vi "0516205_鍾禾翊_HW3.vi"() -> ()   [LabVIEW 2018]
panel:
  in  "Path to JPEG file":path=path "Afu.jpg"
  in  "stop 2":bool
  in  "stop":bool
  out "new picture 5":picture
  in  "Probe":dbl(slide) scale=0.0..10.0
  out "new picture 4":picture
  out "Brighten Image":picture
  out "Original Image":picture
  in  "B 2":u8(slide) scale=0.0..255.0
  in  "G 2":u8(slide) scale=0.0..255.0
  in  "R 2":u8(slide) scale=0.0..255.0
  out "Color Box 2":u32(colorbox)
  out "B":u8(slide) scale=0.0..255.0
  out "G":u8(slide) scale=0.0..255.0
  out "R":u8(slide) scale=0.0..255.0
  in  "Color Box":u32(colorbox)
  # "Color Picker"
  # "Adjust Image Brighteness"
  # "Filter Image with Probe"
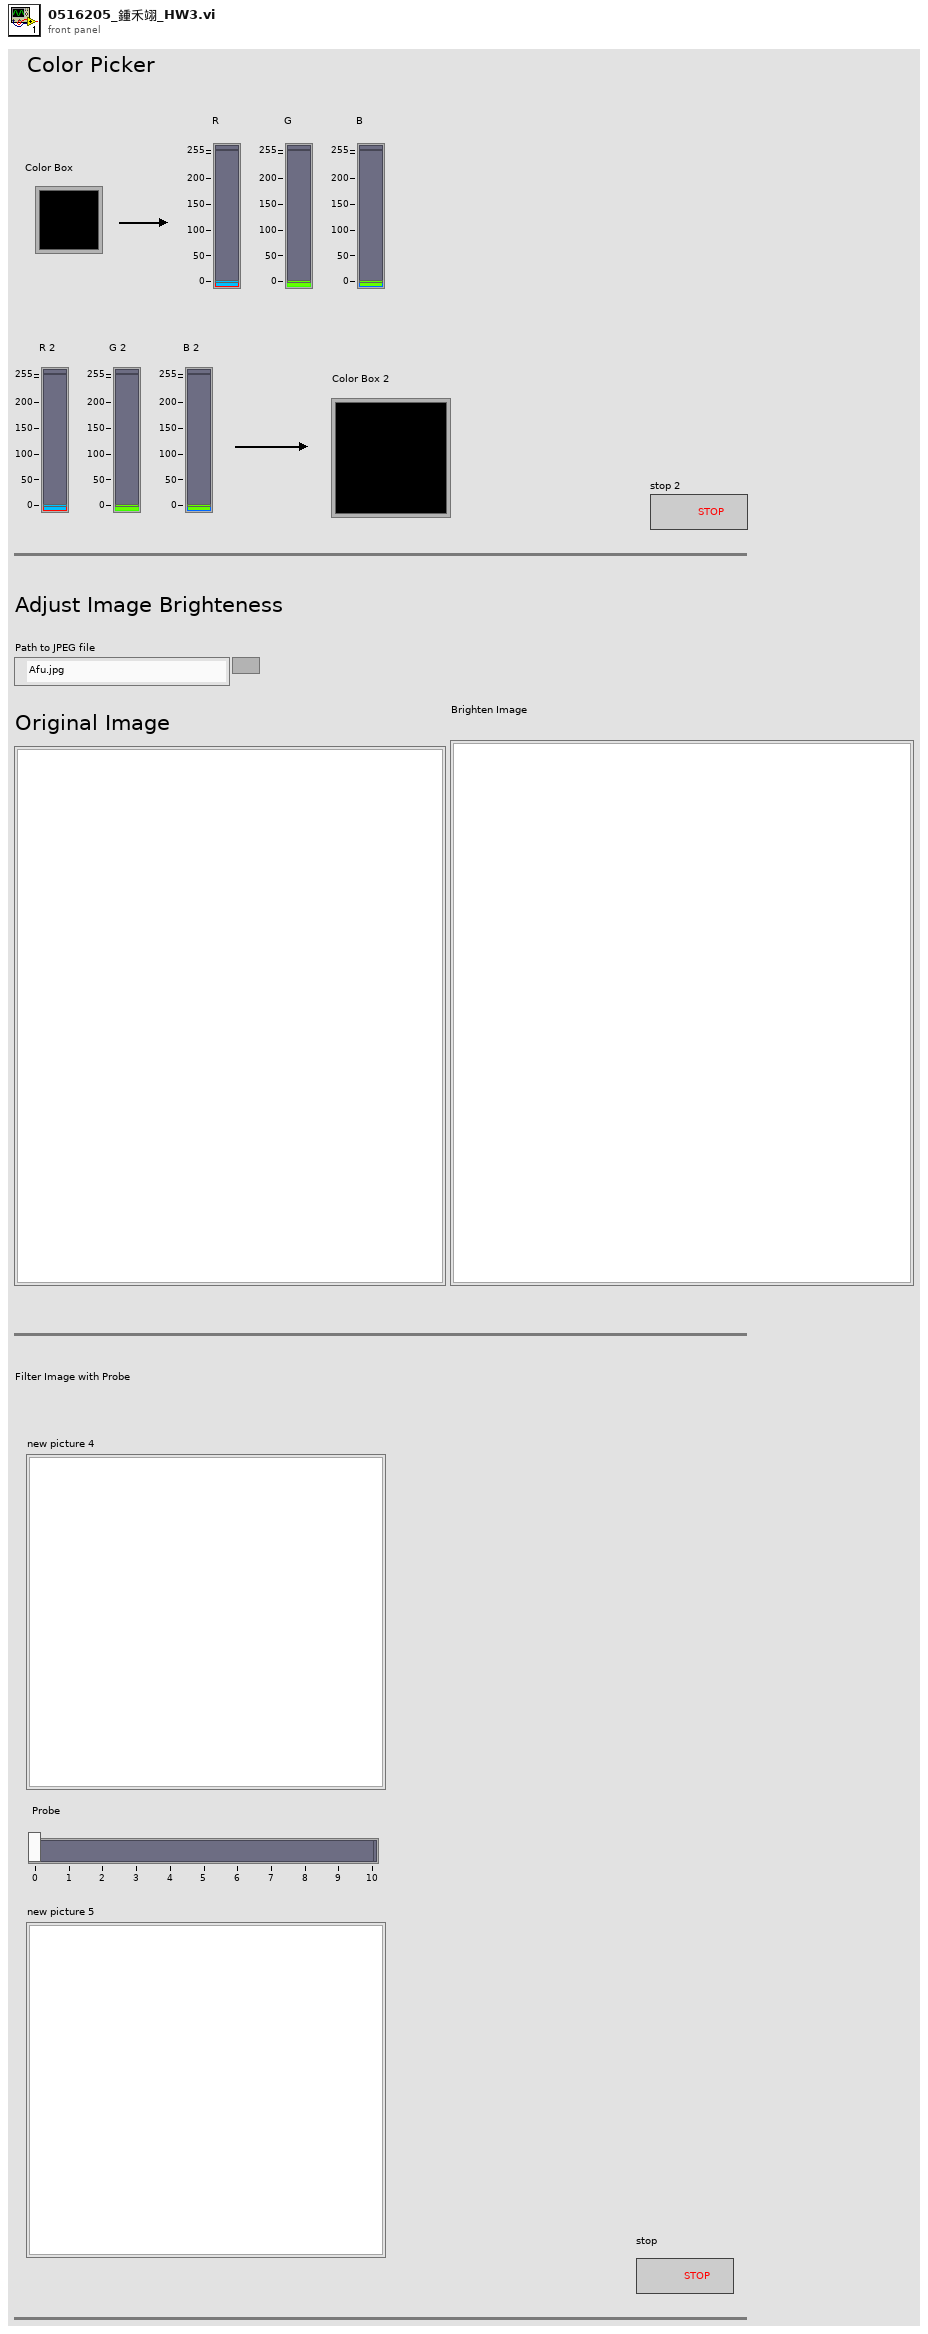
[diagram p1: front panel]
types:
  T1 = typedef "imagedata.ctl" = cluster{"image type":i32, "image depth":i32, "image":u8[], "mask":u8[], "colors":u32[], "Rectangle":cluster{"left":i16, "top":i16, "right":i16, "bottom":i16}}
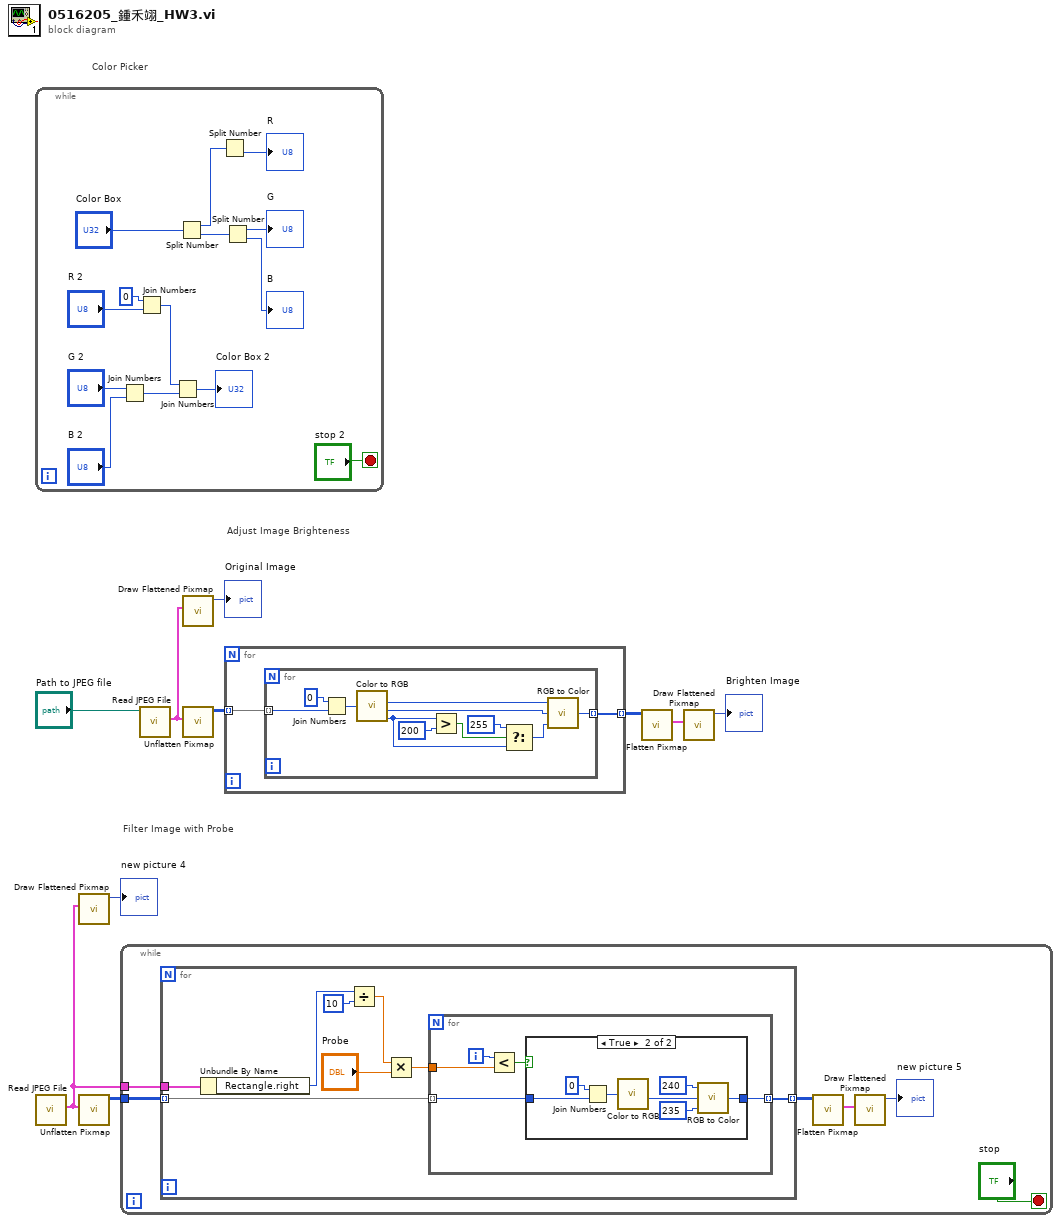
[diagram p0: block diagram]
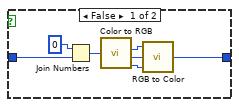
[diagram p2: hidden frame]
diagram:
  # "Filter Image with Probe"
  # "Adjust Image Brighteness"
  # "Color Picker"
  n1 = while {
    stop <- "stop 2" stop-if-true
    n2 = Join Numbers(hi="G 2", lo="B 2") -> ((hi.lo)=w13:u16)
    n3 = Join Numbers(hi=u8 0, lo="R 2") -> ((hi.lo)=w14:u16)
    n4 = Join Numbers(hi=w14, lo=w13) -> ((hi.lo)=→"Color Box 2":u32)
    n5 = Split Number(x="Color Box") -> (hi(x)=w23:u16, lo(x)=w22:u16)
    n6 = Split Number(x=w23) -> (lo(x)=→"R":u8)  [unwired: 1 out]
    n7 = Split Number(x=w22) -> (hi(x)=→"G":u8, lo(x)=→"B":u8)
  }
  n8 = call <vilib>:"Read JPEG File.vi"() -> ("image data"=w2:T1)  [unwired: 9 in, 2 out]
  n9 = call <vilib>:"Draw Flattened Pixmap.vi"("image data"=w2) -> ("new picture"=→"new picture 4":picture)  [unwired: 8 in]
  n10 = call <vilib>:"Unflatten Pixmap.vi"("image data"=w2) -> ("24-bit pixmap"=w3:u32[][])  [unwired: 4 in, 6 out]
  n11 = while {
    tunnel: w3 -> [w30]
    tunnel: w2 -> [w29]
    stop <- "stop" stop-if-true
    n12 = for {
      tunnel: w30 -> [w38] mode=indexing
      tunnel: [w37] -> w27 mode=indexing
      tunnel: w29 -> [w36]
      n13 = Unbundle By Name(w36) -> ("Rectangle.right"=w35:i16)
      n14 = Divide(x=w35, y=10) -> (x/y=w33:dbl)
      n15 = Multiply(x=w33, y="Probe") -> (x*y=w31:dbl)
      n16 = for {
        tunnel: w38 -> [w43] mode=indexing
        tunnel: [w42] -> w37 mode=indexing
        tunnel: w31 -> [w41]
        i -> [w39]
        n17 = Less?(x=w39, y=w41) -> (x < y?=w40:bool)
        n18 = case shown="True" w40 {
          tunnel: w43 -> [w48 w55]
          tunnel: [w44 w54] -> w42
          frame False {
            n19 = Join Numbers(hi=u8 0, lo=w48) -> ((hi.lo)=w49:u64)
            n20 = call <vilib>:"Color to RGB.vi"("Color"=w49) -> ("R"=w47:u8, "G"=w46:u8, "B"=w45:u8)  [unwired: 1 out]
            n21 = call <vilib>:"RGB to Color.vi"("B"=w45, "G"=w46, "R"=w47) -> ("Color"=w44:u32)
          }
          frame True {
            n22 = Join Numbers(hi=u8 0, lo=w55) -> ((hi.lo)=w57:u64)
            n23 = call <vilib>:"Color to RGB.vi"("Color"=w57) -> ("G"=w51:u8)  [unwired: 3 out]
            n24 = call <vilib>:"RGB to Color.vi"("B"=235, "G"=w51, "R"=240) -> ("Color"=w54:u32)
          }
        }
      }
    }
    n25 = call <vilib>:"Flatten Pixmap.vi"("24-bit pixmap"=w27) -> ("image data"=w28:T1)  [unwired: 10 in]
    n26 = call <vilib>:"Draw Flattened Pixmap.vi"("image data"=w28) -> ("new picture"=→"new picture 5":picture)  [unwired: 8 in]
  }
  n27 = call <vilib>:"Read JPEG File.vi"("path to JPEG file"="Path to JPEG file") -> ("image data"=w5:T1)  [unwired: 8 in, 2 out]
  n28 = call <vilib>:"Draw Flattened Pixmap.vi"("image data"=w5) -> ("new picture"=→"Original Image":picture)  [unwired: 8 in]
  n29 = call <vilib>:"Unflatten Pixmap.vi"("image data"=w5) -> ("24-bit pixmap"=w8:u32[][])  [unwired: 4 in, 6 out]
  n30 = for {
    tunnel: w8 -> [w59] mode=indexing
    tunnel: [w58] -> w7 mode=indexing
    n31 = for {
      tunnel: [w63] -> w58 mode=indexing
      tunnel: w59 -> [w69] mode=indexing
      n32 = Join Numbers(hi=u8 0, lo=w69) -> ((hi.lo)=w68:u64)
      n33 = call <vilib>:"Color to RGB.vi"("Color"=w68) -> ("R"=w62:u8, "G"=w61:u8, "B"=w60:u8)  [unwired: 1 out]
      n34 = Greater?(x=w60, y=200) -> (0:w66:bool)
      n35 = Select(t=u8 255, s=w66, f=w60) -> (s? t:f=w64:u8)
      n36 = call <vilib>:"RGB to Color.vi"("B"=w64, "G"=w61, "R"=w62) -> ("Color"=w63:u32)
    }
  }
  n37 = call <vilib>:"Flatten Pixmap.vi"("24-bit pixmap"=w7) -> ("image data"=w6:T1)  [unwired: 10 in]
  n38 = call <vilib>:"Draw Flattened Pixmap.vi"("image data"=w6) -> ("new picture"=→"Brighten Image":picture)  [unwired: 8 in]
